vi "Inline Format.vi"(8 "error in":errorcluster, 11 "VI JSON":string) -> (0 "error out":errorcluster, 3 "Inlined HTML":string)   [LabVIEW 2019]
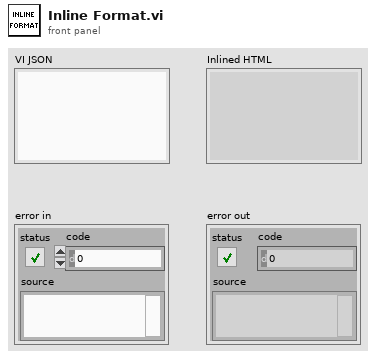
[diagram p1: front panel]
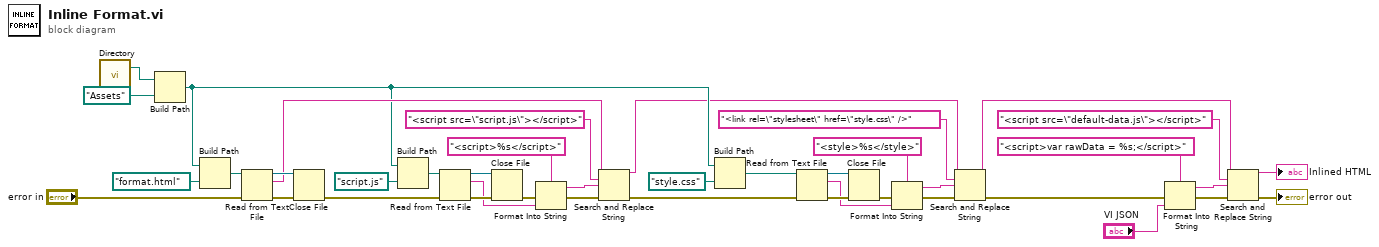
[diagram p0: block diagram]
diagram:
  n1 = call "Directory.vi"() -> ("Directory"=w40:path)  [unwired: 3 in]
  n2 = Build Path(base path=w40, name or relative path=path "Assets") -> (appended path=w23:path)
  n3 = Build Path(base path=w23, name or relative path=path "format.html") -> (appended path=w36:path)
  n4 = Read from Text File(file (use dialog)=w36, error in="error in") -> (refnum out=w38:refnum<file>, text=w26:string, error out=w37:errorcluster)  [unwired: 2 in, 1 out]
  n5 = Close File(refnum=w38, error in=w37) -> (error out=w24:errorcluster)  [unwired: 1 out]
  n6 = Build Path(base path=w23, name or relative path=path "script.js") -> (appended path=w34:path)
  n7 = Read from Text File(file (use dialog)=w34, error in=w24) -> (refnum out=w32:refnum<file>, text=w21:string, error out=w33:errorcluster)  [unwired: 2 in, 1 out]
  n8 = Close File(refnum=w32, error in=w33) -> (error out=w22:errorcluster)  [unwired: 1 out]
  n9 = Format Into String(format string="<script>%s</script>", error in=w22, w21) -> (resulting string=w19:string, error out=w18:errorcluster)  [unwired: 1 in]
  n10 = Search and Replace String(input string=w26, search string="<script src=\"script.js\"></script>", replace string=w19, error in=w18) -> (result string=w5:string, error out=w17:errorcluster)  [unwired: 4 in, 2 out]
  n11 = Build Path(base path=w23, name or relative path=path "style.css") -> (appended path=w27:path)
  n12 = Read from Text File(file (use dialog)=w27, error in=w17) -> (refnum out=w29:refnum<file>, text=w11:string, error out=w28:errorcluster)  [unwired: 2 in, 1 out]
  n13 = Close File(refnum=w29, error in=w28) -> (error out=w12:errorcluster)  [unwired: 1 out]
  n14 = Format Into String(format string="<style>%s</style>", error in=w12, w11) -> (resulting string=w15:string, error out=w16:errorcluster)  [unwired: 1 in]
  n15 = Search and Replace String(input string=w5, search string="<link rel=\"stylesheet\" href=\"style.css\" />", replace string=w15, error in=w16) -> (result string=w1:string, error out=w6:errorcluster)  [unwired: 4 in, 2 out]
  n16 = Format Into String(format string="<script>var rawData = %s;</script>", error in=w6, "VI JSON") -> (resulting string=w9:string, error out=w10:errorcluster)  [unwired: 1 in]
  n17 = Search and Replace String(input string=w1, search string="<script src=\"default-data.js\"></script>", replace string=w9, error in=w10) -> (result string=→"Inlined HTML":string, error out=→"error out":errorcluster)  [unwired: 4 in, 2 out]
